vi "VPCutProjectDependencies.vi"(8 "error in (no error)":errorcluster, 10 "Project In":path) -> (0 "error out":errorcluster, 2 "Temp Project Out":path)   [LabVIEW 2013, in "VIProject.lvlib"]
uses:
  VIProject.lvlib
  <vilib>/xml/Load XML String.vi
  <vilib>/xml/Load XML File.vi
  <vilib>/xml/Close Reference(Node).vi
  <vilib>/xml/Close Reference(NNMap).vi
  <vilib>/xml/NI_XML.lvlib
  <resource>/objmgr/DOMUserDefRef.rc
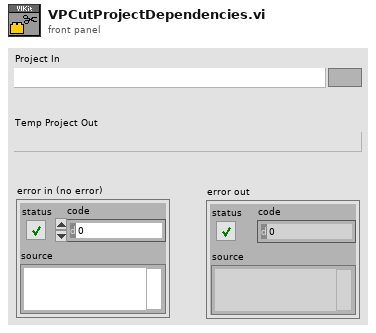
[diagram p1: front panel]
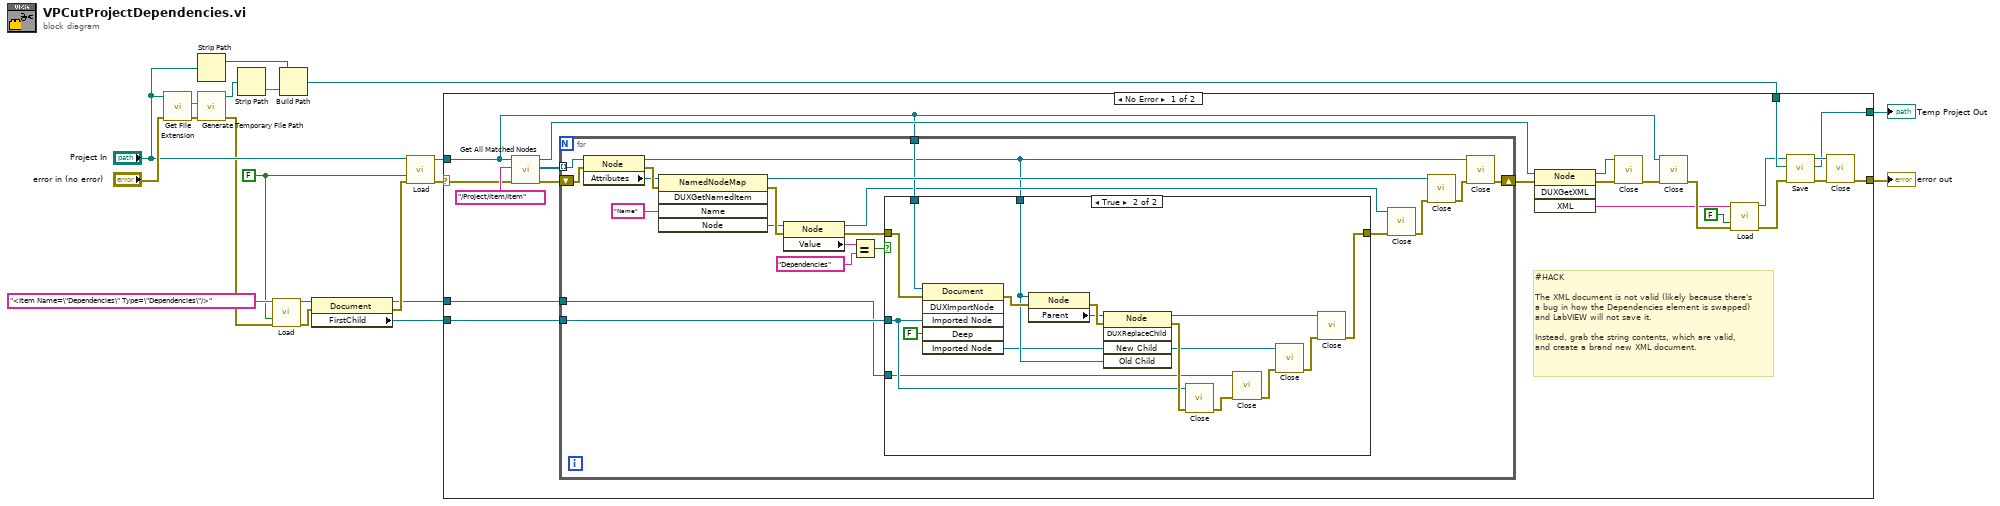
[diagram p0: block diagram]
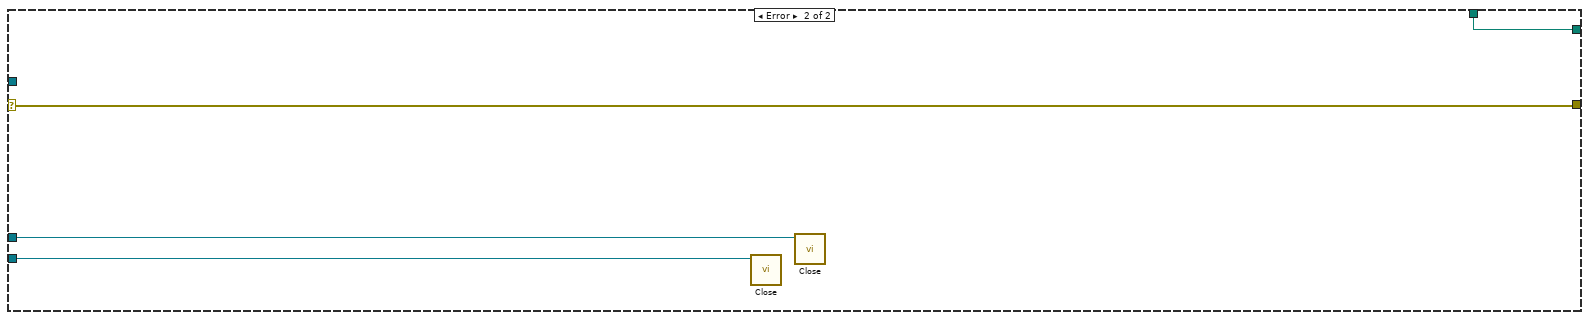
[diagram p3: hidden frame]
diagram:
  w11 = FALSE ("load external DTD (True)")
  n1 = call <vilib>:"Get File Extension.vi"("error in (no error)"="error in (no error)", "file"="Project In") -> ("error out"=w19:errorcluster, "lowercase file extension"=w20:string)  [unwired: 6 in, 2 out]
  n2 = Strip Path(path="Project In") -> (stripped path=w15:path)  [unwired: 1 out]
  n3 = call <vilib>:"Generate Temporary File Path.vi"("error in (no error)"=w19, "Temporary File Extension (tmp)"=w20) -> ("error out"=w6:errorcluster, "Unique Temporary File Path"=w17:path)  [unwired: 8 in]
  n4 = Strip Path(path=w17) -> (name=w16:string)  [unwired: 1 out]
  n5 = call-poly <vilib>:"Load.vi"("XML string"="<Item Name=\"Dependencies\" Type=\"Dependencies\"/>", "load external DTD (True)"=w11, "error in (no error)"=w6) -> ("DOM document out"=w10:refnum<k20>, "error out"=w8:errorcluster)  [unwired: 10 in, 1 out]
  n6 = Build Path(base path=w15, name or relative path=w16) -> (appended path=w13:path)
  n7 = property class="Document"(reference=w10, error in=w8) -> (reference out=w5:refnum<k20>, error out=w7:errorcluster, "FirstChild"=w9:refnum<k20>)
  n8 = call-poly <vilib>:"Load.vi"("path to XML document"="Project In", "load external DTD (True)"=w11, "error in (no error)"=w7) -> ("DOM document out"=w2:refnum<k20>, "error out"=w1:errorcluster)  [unwired: 10 in, 1 out]
  n9 = case shown="No Error" w1 {
    selector: w1 -> [w21 w83]
    tunnel: w13 -> [w42 w84]
    tunnel: w9 -> [w38 w82]
    tunnel: w5 -> [w37 w81]
    tunnel: [w31 w83] -> w4
    tunnel: [w30 w84] -> w3
    tunnel: w2 -> [w27 _]
    frame No Error {
      # "#HACK\n\nThe XML document is not valid (likely because there's a bug in how the Dependencies element is swapped) and LabVIEW will not save it.\n\nInstead, grab the string contents, which are valid, and create a brand new XML document."
      n10 = call <vilib>:"Get All Matched Nodes.vi"("error in (no error)"=w21, "XPath expression"="/Project/Item/Item", "node in"=w27) -> ("error out"=w39:errorcluster, "node result array"=w40:refnum<k20>[], "node out"=w28:refnum<k20>)  [unwired: 6 out]
      n11 = for {
        tunnel: w40 -> [w63] mode=indexing
        tunnel: w38 -> [w49]
        tunnel: w27 -> [w46]
        shift-right: [w55] -> w24
        shift-left: w39 -> [w62]
        tunnel: w37 -> [w45]
        n12 = property class="Node"(reference=w63, error in=w62) -> (reference out=w43:refnum<k20>, error out=w60:errorcluster, "Attributes"=w59:refnum<k20>)
        n13 = invoke class="NamedNodeMap" method="DUXGetNamedItem"(reference=w59, error in=w60, "Name"="Name") -> (reference out=w56:refnum<k20>, error out=w58:errorcluster, "Node"=w57:refnum<k20>)  [unwired: 2 in, 2 out]
        n14 = property class="Node"(reference=w57, error in=w58) -> (reference out=w44:refnum<k20>, error out=w47:errorcluster, "Value"=w53:string)
        n15 = Equal?(x=w53, y="Dependencies") -> (x = y?=w48:bool)
        n16 = case shown="True" w48 {
          tunnel: [w64 w69] -> w50
          tunnel: w49 -> [_ w72]
          tunnel: w47 -> [w64 w76]
          tunnel: w43 -> [_ w74]
          tunnel: w46 -> [_ w78]
          tunnel: w45 -> [_ w68]
          frame False {
          }
          frame True {
            n17 = invoke class="Document" method="DUXImportNode"(reference=w78, error in=w76, "Imported Node"=w72, "Deep"=FALSE) -> (error out=w75:errorcluster, "Imported Node"=w71:refnum<k20>)  [unwired: 2 in, 4 out]
            n18 = property class="Node"(reference=w74, error in=w75) -> (error out=w80:errorcluster, "Parent"=w79:refnum<k20>)  [unwired: 1 out]
            n19 = invoke class="Node" method="DUXReplaceChild"(reference=w79, error in=w80, "New Child"=w71, "Old Child"=w74) -> (reference out=w65:refnum<k20>, error out=w73:errorcluster)  [unwired: 1 in, 3 out]
            n20 = call-poly <vilib>:"Close.vi"("error in (no error)"=w73, "node"=w72) -> ("error out"=w67:errorcluster)  [unwired: 7 out]
            n21 = call-poly <vilib>:"Close.vi"("error in (no error)"=w67, "node"=w68) -> ("error out"=w66:errorcluster)  [unwired: 7 out]
            n22 = call-poly <vilib>:"Close.vi"("error in (no error)"=w66, "node"=w71) -> ("error out"=w70:errorcluster)  [unwired: 7 out]
            n23 = call-poly <vilib>:"Close.vi"("error in (no error)"=w70, "node"=w65) -> ("error out"=w69:errorcluster)  [unwired: 7 out]
          }
        }
        n24 = call-poly <vilib>:"Close.vi"("error in (no error)"=w50, "node"=w44) -> ("error out"=w51:errorcluster)  [unwired: 7 out]
        n25 = call-poly <vilib>:"Close.vi"("error in (no error)"=w51, "named node map"=w56) -> ("error out"=w54:errorcluster)  [unwired: 7 out]
        n26 = call-poly <vilib>:"Close.vi"("error in (no error)"=w54, "node"=w43) -> ("error out"=w55:errorcluster)  [unwired: 7 out]
      }
      n27 = invoke class="Node" method="DUXGetXML"(reference=w28, error in=w24) -> (reference out=w23:refnum<k20>, error out=w25:errorcluster, "XML"=w22:string)  [unwired: 2 in, 1 out]
      n28 = call-poly <vilib>:"Close.vi"("error in (no error)"=w25, "node"=w23) -> ("error out"=w26:errorcluster)  [unwired: 7 out]
      n29 = call-poly <vilib>:"Close.vi"("error in (no error)"=w26, "node"=w27) -> ("error out"=w36:errorcluster)  [unwired: 7 out]
      n30 = call-poly <vilib>:"Load.vi"("XML string"=w22, "load external DTD (True)"=FALSE, "error in (no error)"=w36) -> ("DOM document out"=w34:refnum<k20>, "error out"=w29:errorcluster)  [unwired: 10 in, 1 out]
      n31 = call <vilib>:"Save.vi"("error in (no error)"=w29, "XML file path"=w42, "DOM document in"=w34) -> ("error out"=w33:errorcluster, "XML file path out"=w30:path, "DOM document out"=w32:refnum<k20>)  [unwired: 6 in]
      n32 = call-poly <vilib>:"Close.vi"("error in (no error)"=w33, "node"=w32) -> ("error out"=w31:errorcluster)  [unwired: 7 out]
    }
    frame Error {
      n33 = call-poly <vilib>:"Close.vi"("node"=w82) -> ()  [unwired: 1 in, 8 out]
      n34 = call-poly <vilib>:"Close.vi"("node"=w81) -> ()  [unwired: 1 in, 8 out]
    }
  }
  "Temp Project Out" <- w3
  "error out" <- w4
